vi "Get Desired Size.vi"(8 "error in (no error)":errorcluster, 11 "BP Summary in":refnum<class "BP Summary.lvclass">) -> (0 "error out":errorcluster, 2 "Desired Size":T1={"Width"=0, "Height"=72}, 3 "BP Summary out":refnum<class "BP Summary.lvclass">)   [LabVIEW 2020, in "BP Summary.lvclass"]
uses:
  BP Summary.lvclass
  lv-oopanel/OOPanel/ArrayPanel/Desired Size.ctl
  BP Summary.lvclass/BP Summary.ctl
  BP Item/BP Item.lvclass
  Blueprint/Blueprint.lvclass
  lv-oopanel/OOPanel/ArrayPanel/ArrayPanel.lvclass
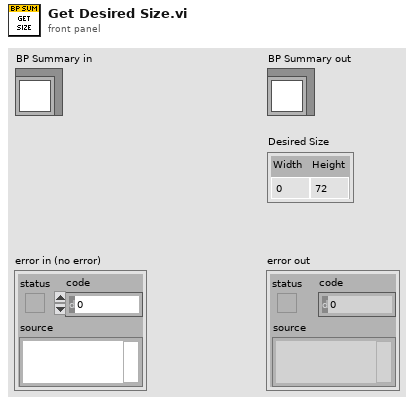
[diagram p1: front panel]
types:
  T1 = typedef "OOPanel.lvlib/ArrayPanel.lvclass/Desired Size.ctl" = cluster{"Width":u32, "Height":u32}
  T2 = typedef "BP Summary.lvclass/Ref Data.ctl" = cluster{"Show Components":bool}
  T3 = typedef "Item.lvclass/Ingredient.ctl" = cluster{"Item":refnum<class "Item.lvclass">, "Qty":dbl}
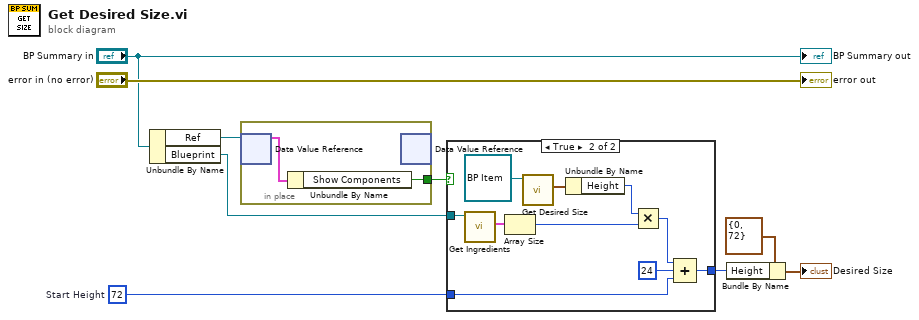
[diagram p0: block diagram]
diagram:
  w9 = u32 72  # Start Height
  n1 = Unbundle By Name("BP Summary in") -> ("Ref"=w4:refnum<data-value>, "Blueprint"=w1:refnum<class "Blueprint.lvclass">)
  n2 = in-place {
    in-place-border: [w10] -> w2
    n3 = in-place-dvr #1(w4) -> (w11:T2)  [unwired: 1 out]
    n4 = Unbundle By Name(w11) -> ("Show Components"=w10:bool)
    n5 = in-place-dvr #1() -> ()  [unwired: 1 in, 2 out]
  }
  n6 = case shown="True" w2 {
    tunnel: w9 -> [w12 w21]
    tunnel: [w12 w20] -> w6
    tunnel: w1 -> [_ w19]
    frame False {
    }
    frame True {
      n7 = call-dynamic "Get Ingredients.vi"("Blueprint in"=w19) -> ("Ingredients"=w18:T3[])  [unwired: 8 in, 2 out]
      n8 = Array Size(array=w18) -> (size(s)=w15:i32)
      n9 = call-dynamic "Get Desired Size.vi"("BP Item in"=refnum<class "BP Item.lvclass"> refnum ("BP Item.lvclass")) -> ("Desired Size"=w16:T1)  [unwired: 8 in, 2 out]
      n10 = Unbundle By Name(w16) -> ("Height"=w14:u32)
      n11 = Multiply(x=w14, y=w15) -> (x*y=w13:u32)
      n12 = Compound Arithmetic op=ADD(w13, u32 24 ("value"), w21) -> (w20:u32)
    }
  }
  n13 = Bundle By Name(cluster=T1 {"Width"=0, "Height"=72} ("Desired Size"), "Height"=w6) -> (→"Desired Size":T1)
  "error out" <- "error in (no error)"
  "BP Summary out" <- "BP Summary in"
